vi "Filter Control Drag Starting Event.vi"(8 "error in (no error)":errorcluster, 10 "ControlDragStartingMsg":refnum<class "ControlDragStartingMsg.lvclass">, 11 "Test Executive Builder Event Filter in":refnum<class "Test Executive Builder Event Filter.lvclass">) -> (0 "error out":errorcluster, 1 "Discard?":bool, 2 "Filtered Event Data":T1, 3 "Test Executive Builder Event Filter out":refnum<class "Test Executive Builder Event Filter.lvclass">, 5 "Data Filtered?":bool)   [LabVIEW 2017, in "Test Executive Builder Event Filter.lvclass"]
uses:
  Test Executive Builder Event Filter.lvclass
  Application Dependencies/Drag Starting Filtered Event Data.ctl
  <vilib>/gpm_packages/@cs/mva-viewable/Source/ActorEvents/IEventAggregator Messages/ControlDragStartingMsg/ControlDragStartingMsg.lvclass
  Test Executive Builder View Messages/Handle Drag Starting Msg/Handle Drag Starting Msg.lvclass
  <vilib>/gpm_packages/@cs/actor-framework-messages/Source/RoundTripMessage/RoundTripMessage.lvclass
  C:/Users/jonmc/Documents/Git/Test Executive Builder/gpm_packages/@cs/actor-framework-messages/Source/RoundTripMessage/RoundTripMessage.lvclass
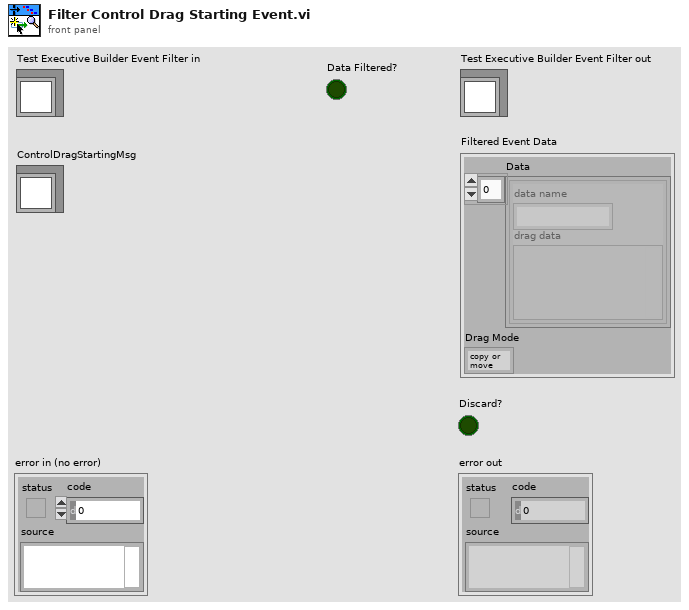
[diagram p1: front panel]
types:
  T1 = cluster{"Data":cluster{"data name":string, "drag data":variant}[], "Drag Mode":enum32{"copy or move", "copy only", "move only"}}
  T2 = typedef "Drag Starting Filtered Event Data.ctl" = cluster{"Drag Mode":enum32{"copy or move", "copy only", "move only"}, "Data Filtered?":bool, "Discard?":bool, "Tag":string, "Dragging?":bool}
  T3 = cluster{"data name":string, "drag data":variant}[]
  T4 = cluster{"Shift":bool, "Ctrl":bool, "Alt":bool, "Cmd":bool, "Opt":bool}
  T5 = typedef "LVPoint32TypeDef.ctl" = cluster{"Horizontal":i32, "Vertical":i32}
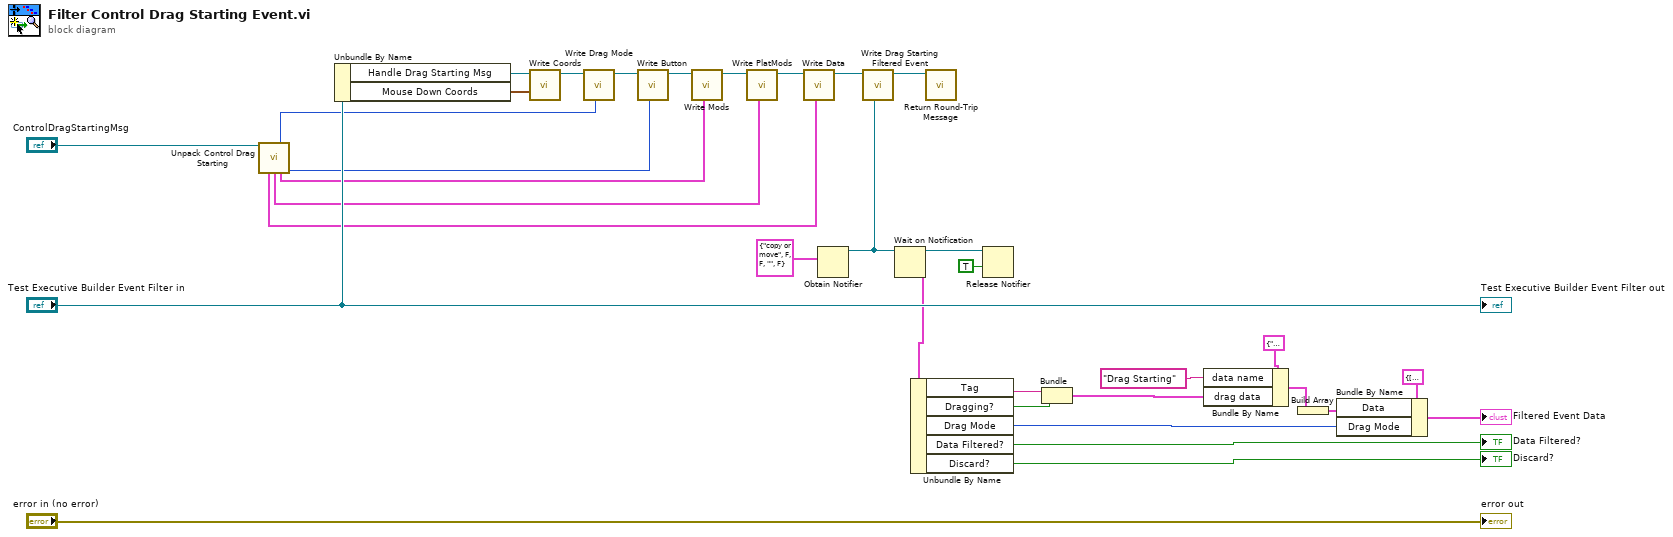
[diagram p0: block diagram]
diagram:
  n1 = call <vilib>:"Unpack Control Drag Starting.vi"("ControlDragStartingMsg In"="ControlDragStartingMsg") -> ("Drag Mode"=w25:enum32{"copy or move", "copy only", "move only"}, "Data"=w17:T3, "PlatMods"=w19:T4, "Mods"=w21:cluster{"Double Click":bool, "Menu Key":bool}, "Button"=w23:u16)  [unwired: 6 in, 4 out]
  n2 = Unbundle By Name("Test Executive Builder Event Filter in") -> ("Handle Drag Starting Msg"=w28:refnum<class "Handle Drag Starting Msg.lvclass">, "Mouse Down Coords"=w27:T5)
  n3 = call "Write Coords.vi"("Coordinates"=w27, "Handle Drag Starting Msg in"=w28) -> ("Handle Drag Starting Msg out"=w26:refnum<class "Handle Drag Starting Msg.lvclass">)  [unwired: 9 in]
  n4 = call "Write Drag Mode.vi"("Drag Mode"=w25, "Handle Drag Starting Msg in"=w26) -> ("Handle Drag Starting Msg out"=w24:refnum<class "Handle Drag Starting Msg.lvclass">)  [unwired: 9 in]
  n5 = call "Write Button.vi"("Button"=w23, "Handle Drag Starting Msg in"=w24) -> ("Handle Drag Starting Msg out"=w22:refnum<class "Handle Drag Starting Msg.lvclass">)  [unwired: 9 in]
  n6 = call "Write Mods.vi"("Mods"=w21, "Handle Drag Starting Msg in"=w22) -> ("Handle Drag Starting Msg out"=w20:refnum<class "Handle Drag Starting Msg.lvclass">)  [unwired: 9 in]
  n7 = call "Write PlatMods.vi"("PlatMods"=w19, "Handle Drag Starting Msg in"=w20) -> ("Handle Drag Starting Msg out"=w18:refnum<class "Handle Drag Starting Msg.lvclass">)  [unwired: 9 in]
  n8 = call "Write Data.vi"("Data"=w17, "Handle Drag Starting Msg in"=w18) -> ("Handle Drag Starting Msg out"=w16:refnum<class "Handle Drag Starting Msg.lvclass">)  [unwired: 9 in]
  n9 = Obtain Notifier(notification data type=T2 {"Drag Mode"=enum."copy or move", "Data Filtered?"=FALSE, "Discard?"=FALSE, "Tag"="", "Dragging?"=FALSE} ("Drag Starting Filtered Event Data")) -> (notifier out=w15:refnum<notifier>)  [unwired: 3 in, 2 out]
  n10 = call "Write Drag Starting Filtered Event.vi"("Drag Starting Filtered Event"=w15, "Handle Drag Starting Msg in"=w16) -> ("Handle Drag Starting Msg out"=w1:refnum<class "Handle Drag Starting Msg.lvclass">)  [unwired: 9 in]
  n11 = Wait on Notification(notifier=w15) -> (notifier out=w32:refnum<notifier>, notification=w14:T2)  [unwired: 3 in, 2 out]
  n12 = Unbundle By Name(w14) -> ("Tag"=w5:string, "Dragging?"=w4:bool, "Drag Mode"=w10:enum32{"copy or move", "copy only", "move only"}, "Data Filtered?"=→"Data Filtered?":bool, "Discard?"=→"Discard?":bool)
  n13 = call <vilib>:"Return Round-Trip Message.vi"("RoundTripMessage In"=w1) -> ()  [unwired: 10 in, 1 out]
  n14 = Release Notifier(notifier=w32, force destroy? (F)=TRUE) -> ()  [unwired: 1 in, 3 out]
  n15 = Bundle("Tag"=w5, "Dragging?"=w4) -> (w3:cluster{"Tag":string, "Dragging?":bool})  [unwired: 1 in]
  n16 = Bundle By Name(cluster=cluster{"data name":string, "drag data":variant} {"data name"="", "drag data"=variant}, "data name"="Drag Starting", "drag data"=w3) -> (w7:cluster{"data name":string, "drag data":variant})
  n17 = Build Array(w7) -> (w6:T3)
  n18 = Bundle By Name(cluster=T1 {"Data"=[], "Drag Mode"=enum."copy or move"} ("Filtered Event Data"), "Data"=w6, "Drag Mode"=w10) -> (→"Filtered Event Data":T1)
  "error out" <- "error in (no error)"
  "Test Executive Builder Event Filter out" <- "Test Executive Builder Event Filter in"
